vi "Do.vi"(8 "error in (no error)":errorcluster, 10 "Actor in":refnum<class "Actor.lvclass">, 11 "SaveCSVImage Msg":refnum<class "SaveCSVImage Msg.lvclass">) -> (0 "error out":errorcluster, 2 "Actor out":refnum<class "Actor.lvclass">)   [LabVIEW 2023, in "InterferometryUI.lvlib" / "SaveCSVImage Msg.lvclass"]
doc: "This VI delivers the message to the actor by calling the appropriate method(s) on the actor."
uses:
  SaveCSVImage Msg.lvclass
  9ef47adc-f318-494c-9b8b-6df3216d6863.vi
  InterferometryUI/InterferometryUI.lvclass
  <vilib>/ActorFramework/Actor/Actor.lvclass
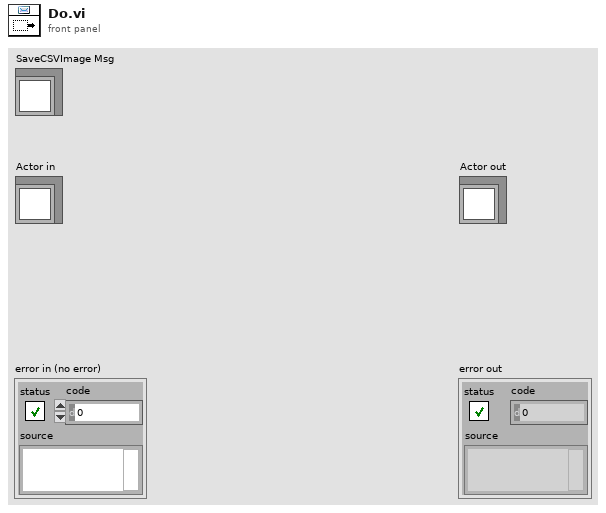
[diagram p1: front panel]
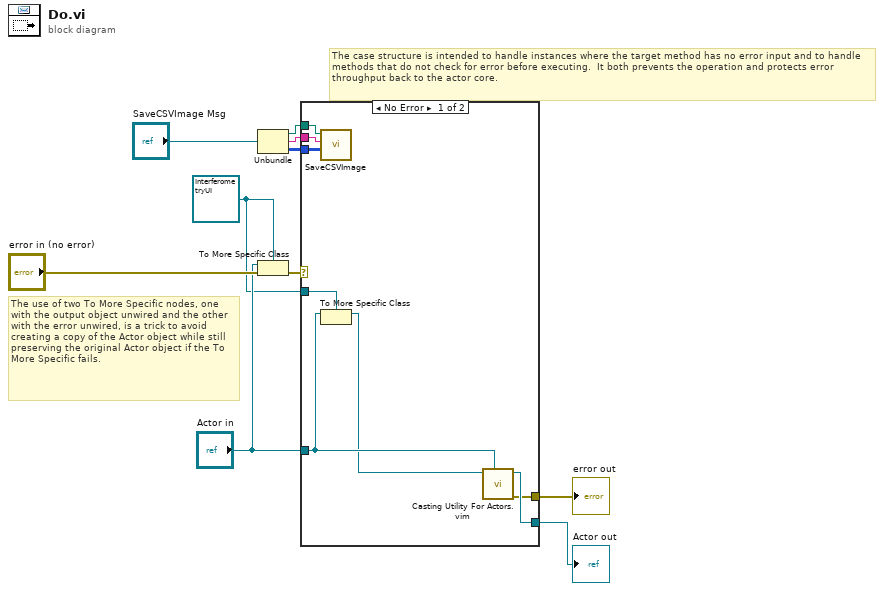
[diagram p0: block diagram]
diagram:
  w4 = refnum<class "InterferometryUI.lvclass"> refnum ("Actor in")
  # "The use of two To More Specific nodes, one with the output object unwired and the other with the error unwired, is a trick to avoid creating a copy of the Actor object while still preserving the original Actor object if the To More Specific fails."
  # "The case structure is intended to handle instances where the target method has no error input and to handle methods that do not check for error before executing.  It both prevents the operation and protects error throughput back to the actor core."
  n1 = Unbundle("SaveCSVImage Msg") -> (w3:path, w2:string, w1:u16[][])
  n2 = To More Specific Class(target class=w4, reference="Actor in", error in="error in (no error)") -> (error out=w8:errorcluster)  [unwired: 1 out]
  n3 = case shown="No Error" w8 {
    selector: w8 -> [_ w20]
    tunnel: [w15 w20] -> w7
    tunnel: [w16 w19] -> w6
    tunnel: "Actor in" -> [w17 w19]
    tunnel: w4 -> [w18 _]
    tunnel: w3 -> [w14 _]
    tunnel: w2 -> [w13 _]
    tunnel: w1 -> [w12 _]
    frame No Error {
      n4 = call "SaveCSVImage.vi"("Image"=w12, "FileName"=w13, "Path"=w14) -> ()  [unwired: 9 in]
      n5 = To More Specific Class(target class=w18, reference=w17) -> (specific class reference=w11:refnum<class "InterferometryUI.lvclass">)  [unwired: 1 in, 1 out]
      n6 = call "Casting Utility For Actors.vim"("type"=w17, "Actor in"=w11) -> ("error out"=w15:errorcluster, "Actor out"=w16:refnum<class "Actor.lvclass">)  [unwired: 8 in]
    }
    frame Error {
      # "If type check fails, pass the original object out again."
    }
  }
  "error out" <- w7
  "Actor out" <- w6
